vi "Read.vi"(8 "error in (no error)":errorcluster, 10 "Bytes to Read (0)":i32, 11 "DeployResource in":refnum<class "Resource.lvclass">) -> (0 "error out":errorcluster, 1 "Bytes Read":i32, 2 "Data":string, 3 "DeployResource out":refnum<class "Resource.lvclass">)   [LabVIEW 2020, in "PicoG-Core.lvlib" / "Resource.lvclass"]
doc: "<b>Bytes to Read</b>:\n -1 to read as many bytes as possible until timeout\n 0 to return current bytes available immediately, ignoring timeout.\n >0 to wait for number of bytes until timeout"
uses:
  Resource.lvclass
  Resource.lvclass/Resource.ctl
  <vilib>/IlluminatedG/lv-stream/stream/Stream.lvclass
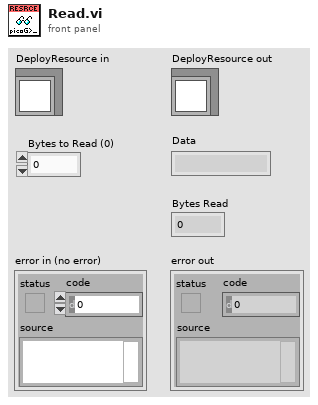
[diagram p1: front panel]
types:
  T1 = typedef "PicoG-Core.lvlib/Resource.lvclass/Ref Data.ctl" = cluster{"Config":map{string, string}, "Client":refnum<class "Connection.lvclass">, "Stream":refnum<class "Stream.lvclass">}
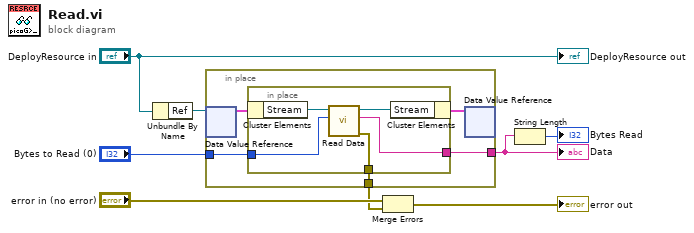
[diagram p0: block diagram]
diagram:
  n1 = Unbundle By Name("DeployResource in") -> ("Ref"=w8:refnum<data-value>)
  n2 = in-place {
    in-place-border: "Bytes to Read (0)" -> [w11]
    in-place-border: [w10] -> w5
    in-place-border: [w9] -> w2
    n3 = in-place-dvr #1(w8) -> (w13:T1)  [unwired: 1 out]
    n4 = in-place {
      in-place-border: w11 -> [w17]
      in-place-border: [w15] -> w10
      in-place-border: [w14] -> w9
      n5 = in-place-cluster #2(w13) -> ("Stream"=w18:refnum<class "Stream.lvclass">)
      n6 = call <vilib>:"Read Data.vi"("Count"=w17, "Stream in"=w18) -> ("error out"=w14:errorcluster, "Data"=w15:string, "Stream out"=w16:refnum<class "Stream.lvclass">)  [unwired: 7 in]
      n7 = in-place-cluster #2("Stream"=w16) -> (w12:T1)
    }
    n8 = in-place-dvr #1(w12) -> ()  [unwired: 2 out]
  }
  "Data" <- w5
  n9 = Merge Errors("error in (no error)", w2) -> (→"error out":errorcluster)
  n10 = String Length(string=w5) -> (length=→"Bytes Read":i32)
  "DeployResource out" <- "DeployResource in"
